vi "Nodos_de_Propiedad_3-Grafica.vi"() -> ()   [LabVIEW 2020]
panel:
  in  "stop":bool
  out "No. Muetreo":i32
  out "Fuera rango":bool
  in  "Lím. Muestreo":i32
  in  "Límite superior":dbl
  in  "T. Muestreo":dbl
  out "String":string
  out "Temperatura":cluster{dbl, "Límite superior":dbl}(graph)
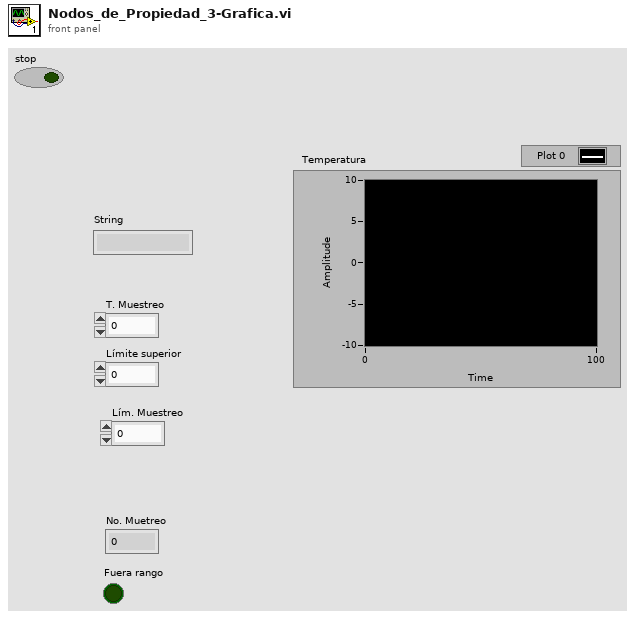
[diagram p1: front panel]
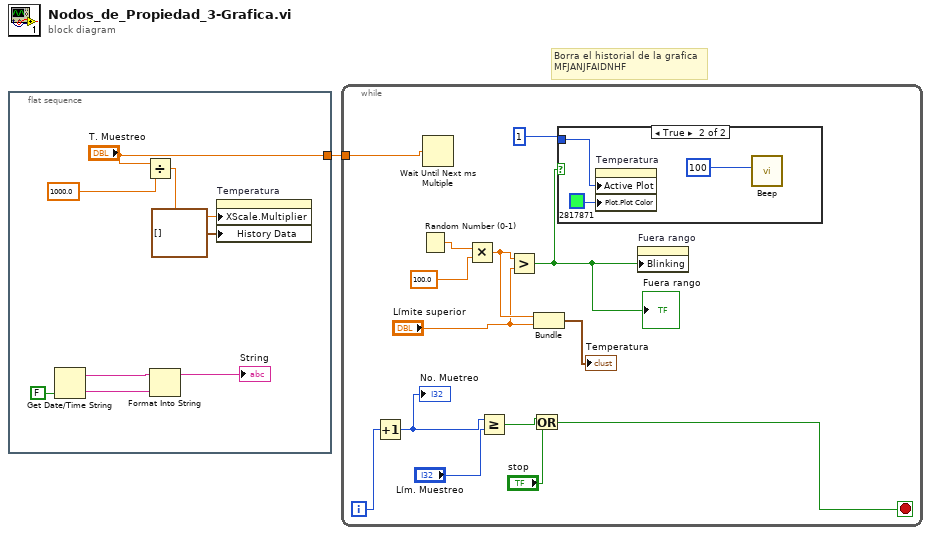
[diagram p0: block diagram]
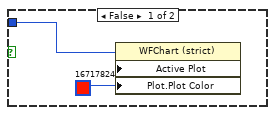
[diagram p2: hidden frame]
diagram:
  # "Borra el historial de la grafica\nMFJANJFAIDNHF"
  n1 = flat-sequence {
    tunnel: ["T. Muestreo"] -> w1
    frame #0 {
      n2 = Get Date/Time String(want seconds? (F)=FALSE) -> (date string=w6:string, time string=w5:string)  [unwired: 2 in]
      n3 = Divide(x="T. Muestreo", y=1000.0) -> (x/y=w8:dbl)
      n4 = Format Into String(initial string=w6, w5) -> (resulting string=→"String":string)  [unwired: 2 in, 1 out]
      n5 = property on="Temperatura" class="WFChart (strict)"("XScale.Multiplier"=w8, "History Data"=cluster{dbl, "Límite superior":dbl}[] []) -> ()  [unwired: 2 in, 2 out]
    }
  }
  n6 = while {
    tunnel: w1 -> [w23]
    i -> [w17]
    stop <- w12 stop-if-true
    n7 = Increment(x=w17) -> (x+1=w15:i32)
    "No. Muetreo" <- w15
    n8 = Random Number (0-1)() -> (number: 0 to 1=w22:dbl)
    n9 = Wait Until Next ms Multiple(millisecond multiple=w23) -> ()  [unwired: 1 out]
    n10 = Multiply(x=w22, y=100.0) -> (x*y=w20:dbl)
    n11 = Greater Or Equal?(x=w15, y="Lím. Muestreo") -> (x >= y?=w14:bool)
    n12 = Greater?(x=w20, y="Límite superior") -> (0:w11:bool)
    "Fuera rango" <- w11
    n13 = Or(x=w14, y="stop") -> (x .or. y?=w12:bool)
    n14 = Bundle(w20, "Límite superior"="Límite superior") -> (→"Temperatura":cluster{dbl, "Límite superior":dbl})  [unwired: 1 in]
    n15 = case shown="True" w11 {
      tunnel: 1 -> [w24 w28]
      frame False {
        n16 = property on="Property Node" class="WFChart (strict)"("Active Plot"=w24, "Plot.Plot Color"=u32 16717824) -> ()  [unwired: 2 in, 2 out]
      }
      frame True {
        n17 = property on="Temperatura" class="WFChart (strict)"("Active Plot"=w28, "Plot.Plot Color"=u32 2817871) -> ()  [unwired: 2 in, 2 out]
        n18 = call <vilib>:"Beep.vi"("duration (msec)"=100) -> ()  [unwired: 11 in]
      }
    }
    n19 = property on="Fuera rango" class="Bool (strict)"("Blinking"=w11) -> ()  [unwired: 2 in, 2 out]
  }
